vi "FTW-Actor-Publish.vi"(0 "FTW-ActorInstance In":refnum<class "FTW-ActorInstance.lvclass">, 5 "Message Header":string, 7 "Message Body":string, 11 "error in (no error)":errorcluster) -> (4 "FTW-ActorInstance Out":refnum<class "FTW-ActorInstance.lvclass">, 15 "error out":errorcluster)   [LabVIEW 2013, in "FTW-ActorInstance.lvclass"]
doc: "This VI has been deprecated and may get removed at any time. DO NOT USE THIS!\n\nIf you need to have a publisher(s) in an actor, add your own publishers to your actor instance. Do not use the base publisher. You have been warned!"
uses:
  FTW-ActorInstance.lvclass
  FTW-ActorInstance.lvclass/FTW-ActorInstance.ctl
  Publisher/FTW-Publisher.lvclass
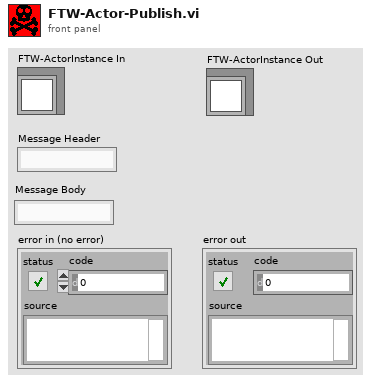
[diagram p1: front panel]
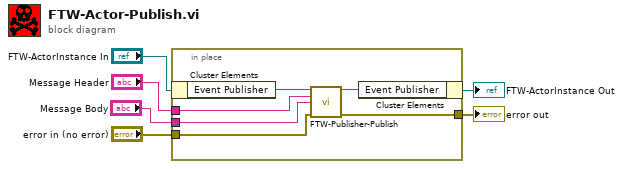
[diagram p0: block diagram]
diagram:
  n1 = in-place {
    in-place-border: "Message Header" -> [w12]
    in-place-border: [w11] -> w5
    in-place-border: "error in (no error)" -> [w10]
    in-place-border: "Message Body" -> [w7]
    n2 = in-place-cluster #1("FTW-ActorInstance In") -> ("Event Publisher"=w9:refnum<class "FTW-Publisher.lvclass">)
    n3 = call "FTW-Publisher-Publish.vi"("FTW-Publisher In"=w9, "Header"=w12, "Body"=w7, "error in"=w10) -> ("FTW-Publisher Out"=w8:refnum<class "FTW-Publisher.lvclass">, "error out"=w11:errorcluster)  [unwired: 10 in]
    n4 = in-place-cluster #1("Event Publisher"=w8) -> (→"FTW-ActorInstance Out":refnum<class "FTW-ActorInstance.lvclass">)
  }
  "error out" <- w5
